vi "PlanMissionPrepMDF.vi"(10 "MDF Array In":T1[](array[typedef]) {"Latitude (waypoint)" format="%#_8g"; "Longitude  (waypoint)" format="%#_8g"}) -> (2 "MDF Array Out":T1[](array[typedef]) {"Latitude (waypoint)" format="%#_8g"; "Longitude  (waypoint)" format="%#_8g"})   [LabVIEW 2010]
uses:
  6-OCU Neurons/MDF LatLong.ctl
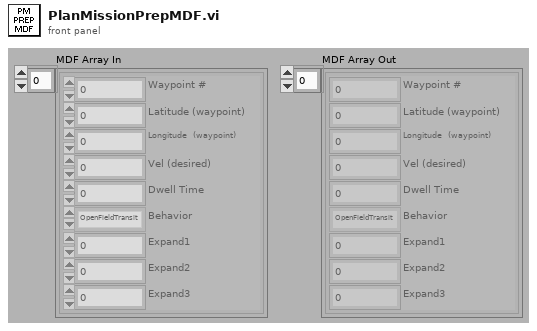
[diagram p1: front panel]
types:
  T1 = typedef "MDF LatLong.ctl" = cluster{"Waypoint #":dbl, "Latitude (waypoint)":ext, "Longitude  (waypoint)":ext, "Vel (desired)":dbl, "Dwell Time":dbl, "Behavior":enum16{"OpenFieldTransit", "WallFollow", "LaneFollow", "ManualMode"}, "Expand1":dbl, "Expand2":dbl, "Expand3":dbl}
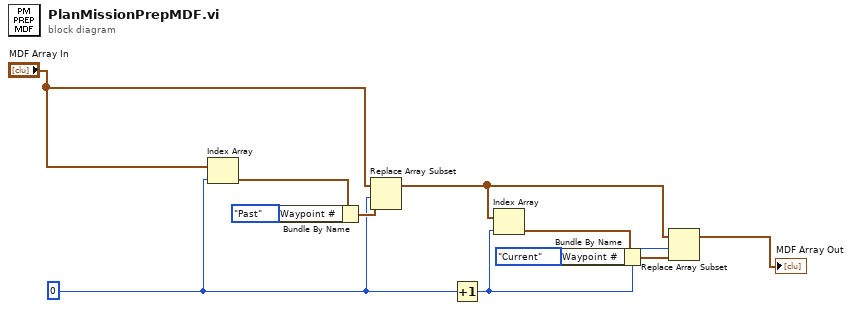
[diagram p0: block diagram]
diagram:
  w8 = i16 0 ("Index")
  n1 = Index Array "Index Array"(array="MDF Array In", index=w8) -> (element=w5:T1)
  n2 = Bundle By Name(cluster=w5, "Waypoint #"=enum16{"Past", "Current", "Future"}."Past" ("Status")) -> (w11:T1)
  n3 = Replace Array Subset "Replace Array Subset"(array="MDF Array In", new element=w11, index=w8) -> (w2:T1[])
  n4 = Increment(x=w8) -> (x+1=w9:i16)
  n5 = Index Array "Index Array"(array=w2, index=w9) -> (element=w3:T1)
  n6 = Bundle By Name(cluster=w3, "Waypoint #"=enum16{"Past", "Current", "Future"}."Current" ("Status")) -> (w10:T1)
  n7 = Replace Array Subset "Replace Array Subset"(array=w2, new element=w10, index=w9) -> (→"MDF Array Out":T1[])
